vi "SSL_get_error.vi"(8 "error in (no error)":errorcluster, 10 "SSL return code":i32, 11 "SSL-Lib in":refnum<class "SSL.lvclass">) -> (0 "error out":errorcluster, 2 "SSL Error Code":T1, 3 "SSL-Lib out":refnum<class "SSL.lvclass">)   [LabVIEW 2013, in "OpenSSL Socket.lvlib" / "SSL.lvclass"]
uses:
  SSL.lvclass
  SSL_Error_Codes.ctl
  SSL-Lib/SSL-Lib.lvclass/SSL-Lib.ctl
  SSL.lvclass/SSL.ctl
  SSL-Lib/Read SSL Library Path.vi
  Read Handle.vi
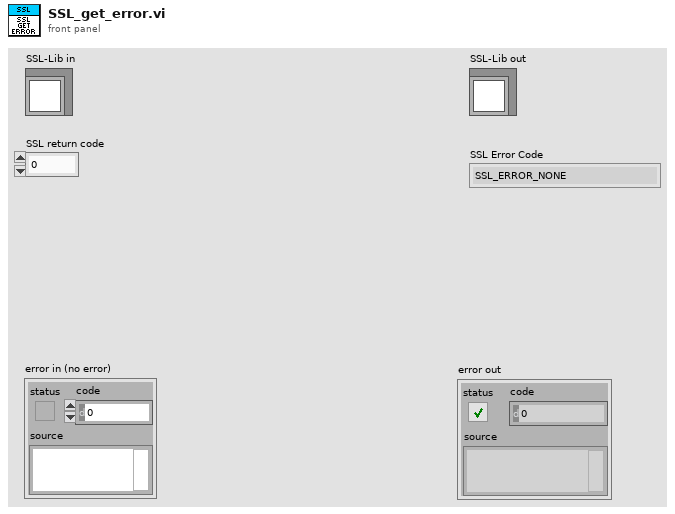
[diagram p1: front panel]
types:
  T1 = typedef "OpenSSL Socket.lvlib/SSL.lvclass/SSL_Error_Codes.ctl" = enum16{"SSL_ERROR_NONE", "SSL_ERROR_SSL", "SSL_ERROR_WANT_READ", "SSL_ERROR_WANT_WRITE", "SSL_ERROR_WANT_X509_LOOKUP", "SSL_ERROR_SYSCALL", "SSL_ERROR_ZERO_RETURN", "SSL_ERROR_WANT_CONNECT", "SSL_ERROR_WANT_ACCEPT"}
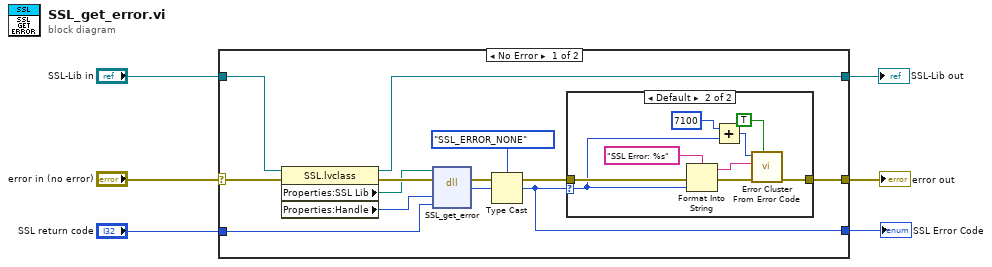
[diagram p0: block diagram]
diagram:
  n1 = case shown="No Error" "error in (no error)" {
    selector: "error in (no error)" -> [w18 w29]
    tunnel: [w13 w30] -> w4
    tunnel: "SSL-Lib in" -> [w12 w30]
    tunnel: "SSL return code" -> [w17 _]
    tunnel: [w9 w29] -> w2
    tunnel: [w7 _] -> w1
    frame No Error {
      n2 = property class="SSL.lvclass"(reference=w12, error in=w18) -> (reference out=w13:refnum<class "SSL.lvclass">, error out=w16:errorcluster, "Properties:SSL Lib"=w15:path, "Properties:Handle"=w14:u64)
      n3 = dll-call lib="C:/Program Files (x86)/National Instruments/Shared/nissl/NIssleay32.dll" fn="SSL_get_error"(path in=w15, error in=w16, "SSL"=w14, "ret"=w17) -> (error out=w10:errorcluster, "return type"=w11:u32)  [unwired: 3 in, 1 out]
      n4 = Type Cast(type=SSL_Error_Codes."SSL_ERROR_NONE" ("SSL Error"), x=w11) -> (*(type *) &x=w7:T1)
      n5 = case shown="Default" w7 {
        selector: w7 -> [_ w23]
        tunnel: w10 -> [w19 w28]
        tunnel: [w19 w27] -> w9
        frame "SSL_ERROR_NONE" {
        }
        frame Default {
          n6 = Format Into String(format string="SSL Error: %s", error in=w28, w23) -> (resulting string=w22:string, error out=w24:errorcluster)  [unwired: 1 in]
          n7 = Add(x=7100, y=w23) -> (x+y=w26:i32)
          n8 = call <vilib>:"Error Cluster From Error Code.vi"("show call chain? (False)"=TRUE, "error in (no error)"=w24, "error message (\"\")"=w22, "error code (0)"=w26) -> ("error out"=w27:errorcluster)  [unwired: 5 in]
        }
      }
    }
    frame Error {
    }
  }
  "SSL-Lib out" <- w4
  "error out" <- w2
  "SSL Error Code" <- w1
